vi "IMAQ FPGA Image Transfer from Target U64.vi"(7 "Read Timeout (ms)":i32=5000, 8 "error in (no error)":errorcluster, 9 "DMA FIFO Reference In":refnum<k20>, 10 "Maximum Pixels per Read":i32=-1, 11 "Image":T1) -> (0 "error out":errorcluster, 1 "DMA FIFO Reference Out":refnum<k20>, 3 "Image Out":T1)   [LabVIEW 2017, in "NI_VDM_FPGA_Basics.lvlib"]
doc: "Transfers an image from the target FPGA to the host processor via DMA FIFO."
uses:
  <vilib>/visionFPGA/NI_VDM_FPGA_Basics.lvlib
  <vilib>/vision/Image Controls.llb/IMAQ Image.ctl
  <vilib>/rvi/errors/niLvFpgaAdjustHostInterfaceError.vi
  <vilib>/rvi/interface/nirviMethod/nirviMethod.xnode
  <vilib>/rvi/errors/niLvFpgaMergeErrorWithErrorCode.vi
  <vilib>/FPGAPlugInAG/Dynamic/niLvFpga_ReadFifo_Dynamic.vi
  <vilib>/FPGAPlugInAG/Dynamic/niLvFpga_AcquireReadRegionFifo_Dynamic.vi
  <vilib>/vision/EDVR.llb/IMAQ ImageToEDVR 2D U64.vi
  nivissvc.dll
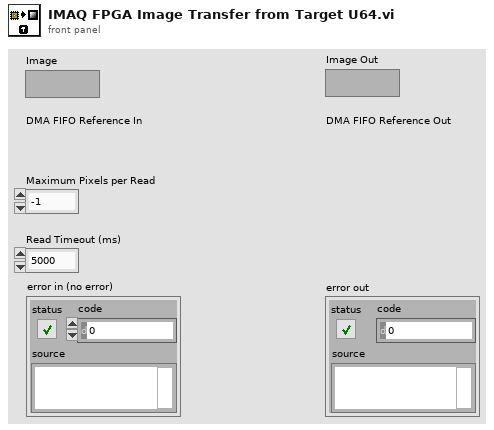
[diagram p1: front panel]
types:
  T1 = typedef "IMAQ Image.ctl" = refnum<image>
  T2 = typedef "Image Type" = u32
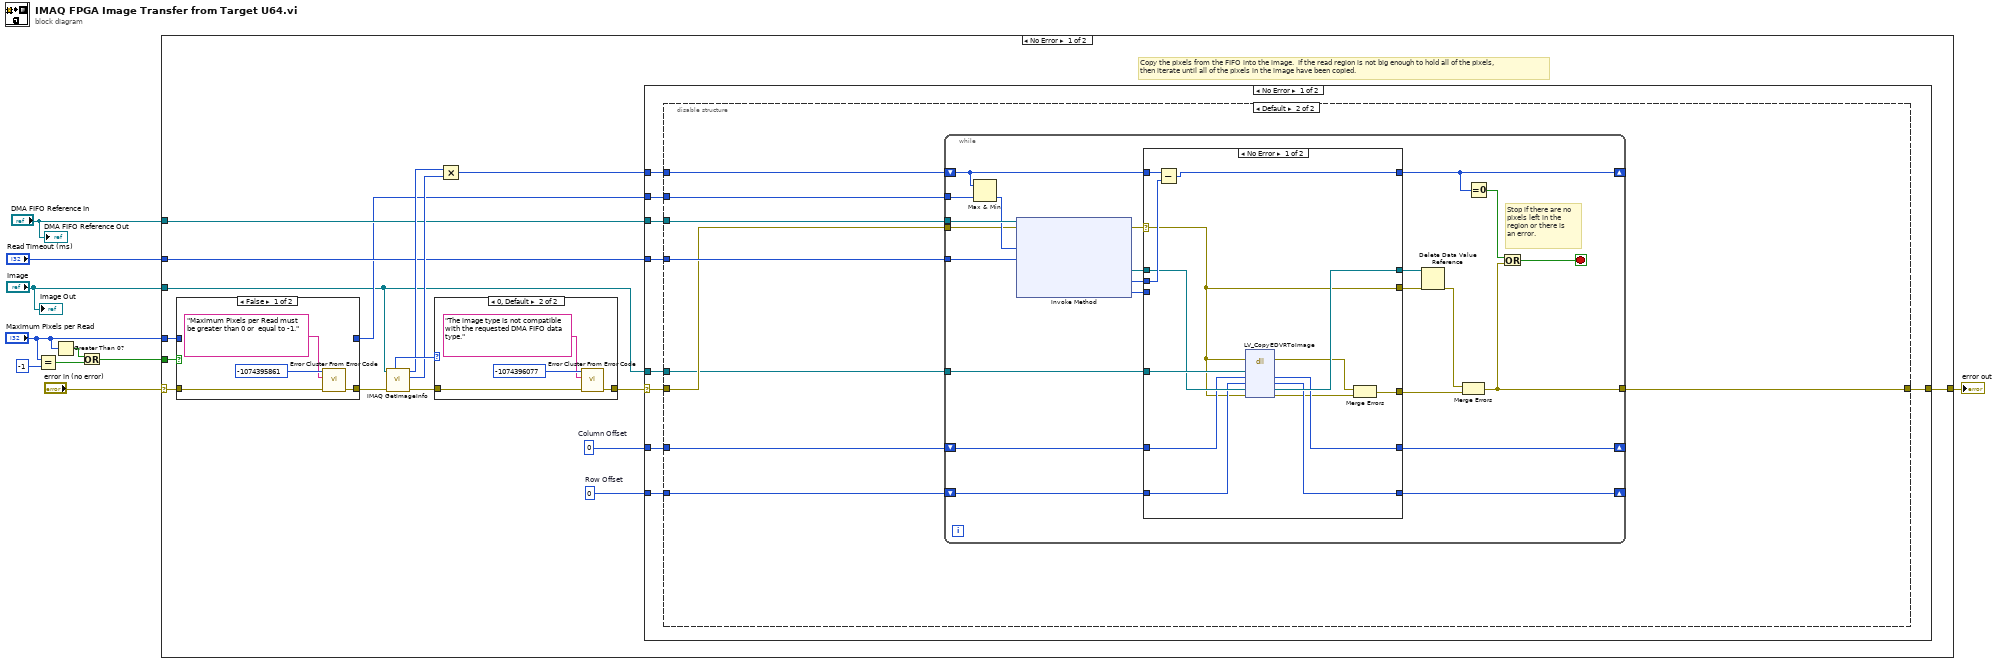
[diagram p0: block diagram]
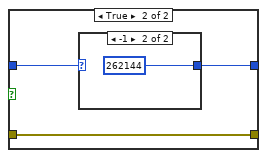
[diagram p2: hidden frame]
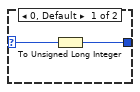
[diagram p3: hidden frame]
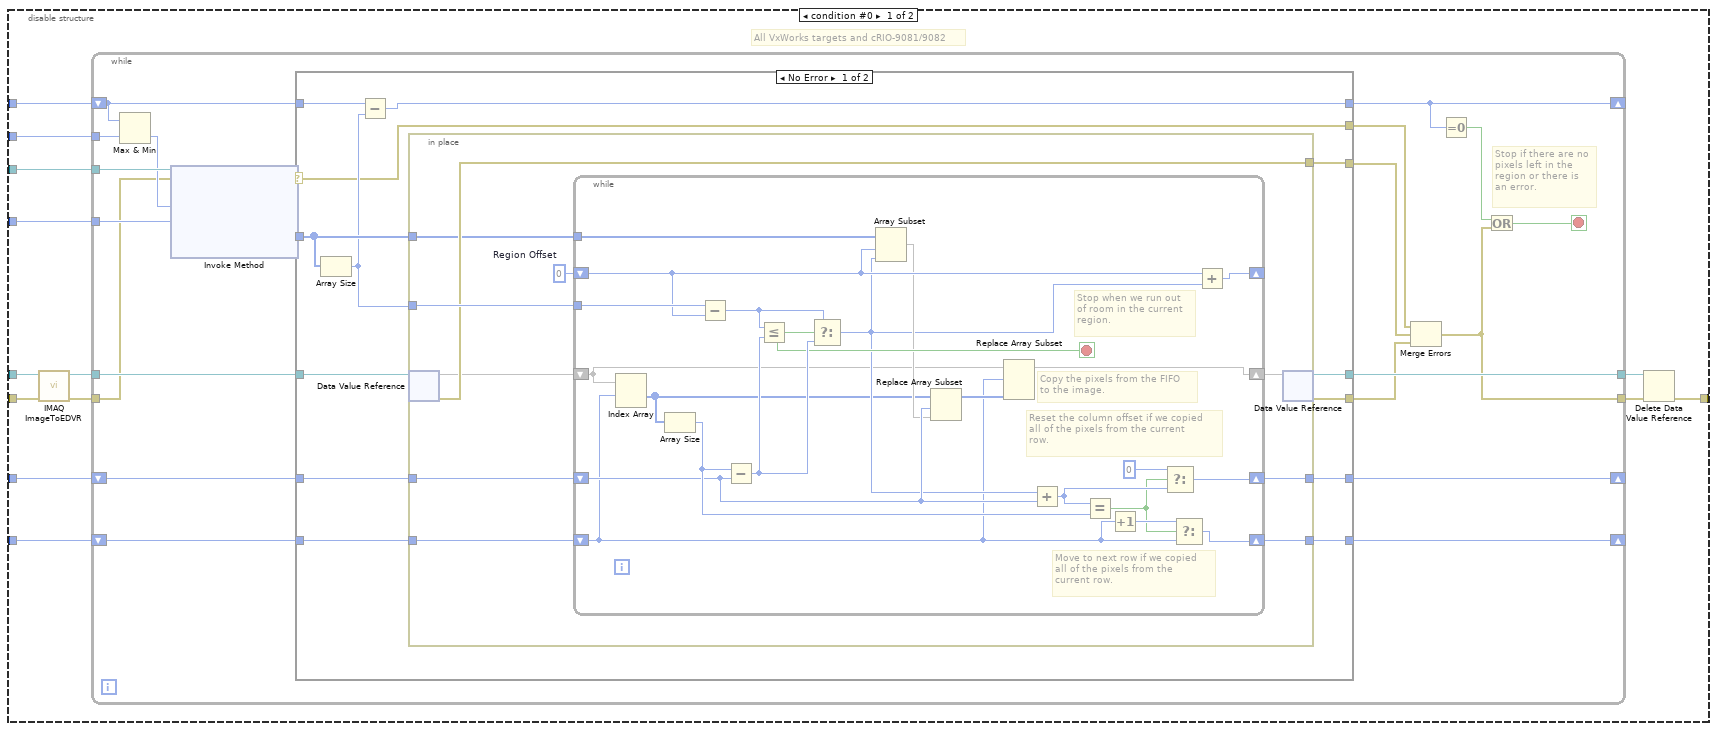
[diagram p4: hidden frame]
diagram:
  n1 = Equal?(x="Maximum Pixels per Read", y=-1) -> (x = y?=w6:bool)
  n2 = Greater Than 0?(x="Maximum Pixels per Read") -> (x > 0?=w7:bool)
  n3 = Or(x=w7, y=w6) -> (x .or. y?=w5:bool)
  n4 = case shown="No Error" "error in (no error)" {
    selector: "error in (no error)" -> [w11 w188]
    tunnel: "DMA FIFO Reference In" -> [w22 _]
    tunnel: "Read Timeout (ms)" -> [w21 _]
    tunnel: w5 -> [w18 _]
    tunnel: "Maximum Pixels per Read" -> [w16 _]
    tunnel: "Image" -> [w13 _]
    tunnel: [w12 w188] -> w2
    frame No Error {
      w19 = u32 0  # Row Offset
      w20 = u32 0  # Column Offset
      # "Copy the pixels from the FIFO into the image.  If the read region is not big enough to hold all of the pixels,\nthen iterate until all of the pixels in the image have been copied."
      n5 = case shown="False" w18 {
        tunnel: w11 -> [w29 w34]
        tunnel: [w28 w34] -> w17
        tunnel: w16 -> [_ w33]
        tunnel: [_ w32] -> w15
        frame False {
          n6 = call <vilib>:"Error Cluster From Error Code.vi"("error in (no error)"=w29, "error message (\"\")"="Maximum Pixels per Read must be greater than 0 or  equal to -1." ("error message (\"\")"), "error code (0)"=-1074395861) -> ("error out"=w28:errorcluster)  [unwired: 6 in]
        }
        frame True {
          n7 = case shown="-1" w33 {
            selector: w33 -> [w36 _]
            tunnel: [w35 u32 262144 ("Maximum Pixels per Write")] -> w32
            frame 0, Default {
              n8 = To Unsigned Long Integer(number=w36) -> (unsigned 32bit integer=w35:u32)
            }
            frame -1 {
            }
          }
        }
      }
      n9 = call "IMAQ GetImageInfo"("error in (no error)"=w17, "Image"=w13) -> ("error out"=w26:errorcluster, "Y Resolution"=w24:i32, "X Resolution"=w25:i32, "Image Type"=w27:T2)  [unwired: 2 in, 4 out]
      n10 = case shown="0, Default" w27 {
        tunnel: w26 -> [w183 w185]
        tunnel: [w183 w184] -> w14
        frame 6 {
          # "Allowed types are:\nRGB (U64)"
        }
        frame 0, Default {
          n11 = call <vilib>:"Error Cluster From Error Code.vi"("error in (no error)"=w185, "error message (\"\")"="The image type is not compatible with the requested DMA FIFO data type." ("error message (\"\")"), "error code (0)"=-1074396077) -> ("error out"=w184:errorcluster)  [unwired: 6 in]
        }
      }
      n12 = Multiply(x=w25, y=w24) -> (x*y=w23:i32)
      n13 = case shown="No Error" w14 {
        selector: w14 -> [w41 w182]
        tunnel: w23 -> [w46 _]
        tunnel: w20 -> [w40 _]
        tunnel: w19 -> [w39 _]
        tunnel: w22 -> [w44 _]
        tunnel: [w38 w182] -> w12
        tunnel: w15 -> [w45 _]
        tunnel: w21 -> [w43 _]
        tunnel: w13 -> [w42 _]
        frame No Error {
          n14 = disable-structure shown="Default" {
            disable-tunnel: w46 -> [w59 w139]
            disable-tunnel: w40 -> [w58 w138]
            disable-tunnel: w39 -> [w57 w137]
            disable-tunnel: w44 -> [w56 w136]
            disable-tunnel: [w47 w135] -> w38
            disable-tunnel: w45 -> [w55 w134]
            disable-tunnel: w43 -> [w54 w133]
            disable-tunnel: w42 -> [w53 w131]
            disable-tunnel: w41 -> [w51 w132]
            frame condition #0 {
              # "All VxWorks targets and cRIO-9081/9082"
              n15 = call-poly <vilib>:"IMAQ ImageToEDVR.vi"("error in (no error)"=w51, "Image"=w53) -> ("error out"=w50:errorcluster, "EDVR 2D U64"=w52:refnum<data-value>)  [unwired: 7 in, 1 out]
              n16 = while {
                shift-right: [w71] -> _
                shift-left: w59 -> [w67]
                shift-right: [w76] -> _
                shift-left: w58 -> [w78]
                shift-right: [w79] -> _
                shift-left: w57 -> [w77]
                tunnel: w56 -> [w75]
                tunnel: [w73] -> w49
                tunnel: [w69] -> w48
                tunnel: w55 -> [w65]
                tunnel: w54 -> [w64]
                tunnel: w52 -> [w61]
                tunnel: w50 -> [w60]
                stop <- w70 stop-if-true
                # "Stop if there are no\npixels left in the \nregion or there is\nan error."
                n17 = Max & Min(x=w67, y=w65) -> (min(x,y)=w66:u32)  [unwired: 1 out]
                n18 = xnode "Invoke Method"("FPGA VI Reference In"=w75, "error in"=w60, "Number of Elements"=w66, "Timeout (ms)"=w64) -> ("error out"=w74:errorcluster, "Data"=w80:u64[])  [unwired: 2 out]
                n19 = case shown="No Error" w74 {
                  selector: w74 -> [w81 w126]
                  tunnel: w67 -> [w93 w129]
                  tunnel: [w92 w129] -> w71
                  tunnel: w61 -> [w91 w130]
                  tunnel: w80 -> [w83 _]
                  tunnel: [w90 w127] -> w79
                  tunnel: w78 -> [w89 w128]
                  tunnel: w77 -> [w88 w127]
                  tunnel: [w87 w128] -> w76
                  tunnel: [w86 w130] -> w73
                  tunnel: [w81 w126] -> w63
                  tunnel: [w85 _] -> w62
                  tunnel: [w84 _] -> w72
                  frame No Error {
                    n20 = Array Size(array=w83) -> (size(s)=w82:i32)
                    n21 = Subtract(x=w93, y=w82) -> (x-y=w92:i32)
                    n22 = in-place {
                      in-place-border: w82 -> [w101]
                      in-place-border: [w103] -> w90
                      in-place-border: w89 -> [w100]
                      in-place-border: w88 -> [w96]
                      in-place-border: [w99] -> w87
                      in-place-border: [w98] -> w84
                      in-place-border: w83 -> [w94]
                      w102 = u32 0  # Region Offset
                      n23 = in-place-dvr #1(w91) -> (w97:u64[][], w98:errorcluster)
                      n24 = while {
                        shift-right: [w123] -> _
                        shift-left: w102 -> [w122]
                        tunnel: w94 -> [w112]
                        tunnel: w101 -> [w125]
                        shift-right: [w117] -> w99
                        shift-left: w100 -> [w113]
                        shift-right: [w104] -> w95
                        shift-left: w97 -> [w107]
                        shift-right: [w115] -> w103
                        shift-left: w96 -> [w105]
                        stop <- w114 stop-if-true
                        # "Stop when we run out\nof room in the current\nregion."
                        # "Copy the pixels from the FIFO\nto the image."
                        # "Reset the column offset if we copied\nall of the pixels from the current\nrow."
                        # "Move to next row if we copied\nall of the pixels from the\ncurrent row."
                        n25 = Index Array(array=w107, index (row)=w105) -> (element=w108:u64[])  [unwired: 1 in]
                        n26 = Array Size(array=w108) -> (size(s)=w121:i32)
                        n27 = Subtract(x=w125, y=w122) -> (x-y=w124:u32)
                        n28 = Subtract(x=w121, y=w113) -> (x-y=w120:u32)
                        n29 = Less Or Equal?(x=w124, y=w120) -> (x <= y?=w114:bool)
                        n30 = Select(t=w124, s=w114, f=w120) -> (s? t:f=w110:u32)
                        n31 = Array Subset(array=w112, index=w122, length=w110) -> (w111:u64[])
                        n32 = Replace Array Subset(array=w108, new element=w111, index=w113) -> (w106:u64[])
                        n33 = Replace Array Subset(array=w107, new element=w106, index (row)=w105) -> (w104:u64[][])  [unwired: 1 in]
                        n34 = Add(x=w110, y=w113) -> (x+y=w118:u32)
                        n35 = Equal?(x=w118, y=w121) -> (x = y?=w109:bool)
                        n36 = Increment(x=w105) -> (x+1=w116:u32)
                        n37 = Select(t=u32 0 ("Elements In Region"), s=w109, f=w118) -> (s? t:f=w117:u32)
                        n38 = Select(t=w116, s=w109, f=w105) -> (s? t:f=w115:u32)
                        n39 = Add(x=w122, y=w110) -> (x+y=w123:u32)
                      }
                      n40 = in-place-dvr #1(w95) -> (w86:refnum<data-value>, w85:errorcluster)
                    }
                  }
                  frame Error {
                  }
                }
                n41 = Merge Errors(w63, w72, w62) -> (w69:errorcluster)
                n42 = Equal To 0?(x=w71) -> (x = 0?=w68:bool)
                n43 = Or(x=w68, y=w69) -> (x .or. y?=w70:bool)
              }
              n44 = Delete Data Value Reference(data value reference=w49, error in=w48) -> (error out=w47:errorcluster)  [unwired: 1 out]
            }
            frame condition #1 (active) {
              n45 = while {
                shift-right: [w153] -> _
                shift-left: w139 -> [w150]
                shift-right: [w157] -> _
                shift-left: w138 -> [w159]
                shift-right: [w160] -> _
                shift-left: w137 -> [w158]
                tunnel: w136 -> [w156]
                tunnel: [w140] -> w135
                tunnel: w134 -> [w147]
                tunnel: w133 -> [w146]
                tunnel: w132 -> [w145]
                tunnel: w131 -> [w144]
                stop <- w152 stop-if-true
                # "Stop if there are no\npixels left in the \nregion or there is\nan error."
                n46 = Max & Min(x=w150, y=w147) -> (min(x,y)=w149:u32)  [unwired: 1 out]
                n47 = xnode "Invoke Method"("FPGA VI Reference In"=w156, "error in"=w145, "Number of Elements"=w149, "Timeout (ms)"=w146) -> ("error out"=w155:errorcluster, "Read Region Reference"=w162:refnum<data-value>, "Elements In Region"=w161:u32, "Elements Remaining"=w148:u32)  [unwired: 1 out]
                n48 = case shown="No Error" w155 {
                  selector: w155 -> [w163 w177]
                  tunnel: w150 -> [w176 w181]
                  tunnel: [w175 w181] -> w153
                  tunnel: w162 -> [w171 w178]
                  tunnel: w161 -> [w172 _]
                  tunnel: [w167 w179] -> w160
                  tunnel: w159 -> [w170 w180]
                  tunnel: w158 -> [w169 w179]
                  tunnel: [w168 w180] -> w157
                  tunnel: [w173 w178] -> w154
                  tunnel: [w163 w177] -> w143
                  tunnel: w148 -> [_ _]
                  tunnel: w144 -> [w174 _]
                  tunnel: [w164 w177] -> w142
                  frame No Error {
                    n49 = Subtract(x=w176, y=w172) -> (x-y=w175:u32)
                    n50 = dll-call lib="nivissvc.*" fn="LV_CopyEDVRToImage"(error in=w163, "image"=w174, "xImageOffset"=w170, "yImageOffset"=w169, "EDVR"=w171, "error"=w163) -> (error out=w165:errorcluster, "xImageOffset"=w168:u32, "yImageOffset"=w167:u32, "EDVR"=w173:refnum<data-value>, "error"=w166:errorcluster)  [unwired: 4 in, 1 out]
                    n51 = Merge Errors(w165, w166) -> (w164:errorcluster)
                  }
                  frame Error {
                  }
                }
                n52 = Delete Data Value Reference(data value reference=w154, error in=w143) -> (error out=w141:errorcluster)  [unwired: 1 out]
                n53 = Merge Errors(w141, w142) -> (w140:errorcluster)
                n54 = Equal To 0?(x=w153) -> (x = 0?=w151:bool)
                n55 = Or(x=w151, y=w140) -> (x .or. y?=w152:bool)
              }
            }
          }
        }
        frame Error {
        }
      }
    }
    frame Error {
    }
  }
  "error out" <- w2
  "Image Out" <- "Image"
  "DMA FIFO Reference Out" <- "DMA FIFO Reference In"
